vi "fn Browse Server.vi"(8 "error in (no error)":errorcluster) -> (0 "error out":errorcluster, 3 "[Items]":string[](array[string]))   [LabVIEW 2018, in "LV_OPC.lvlib"]
doc: "LVOPC_API int fnBrowseServer(char* LV_items[]);"
uses:
  LV_OPC.lvlib
  LVOPC64.dll
panel:
  out "LV_items out":string
  out "function return":i32
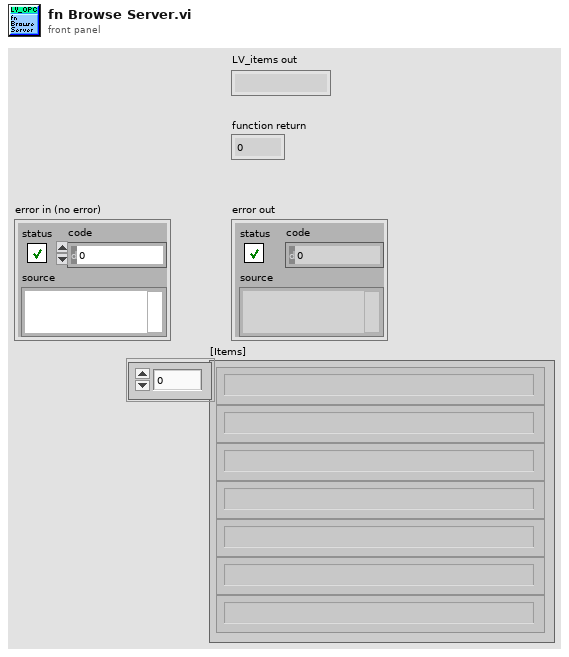
[diagram p1: front panel]
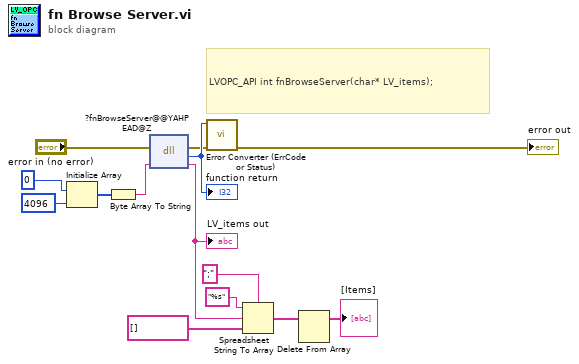
[diagram p0: block diagram]
diagram:
  # "LVOPC_API int fnBrowseServer(char* LV_items);"
  n1 = Initialize Array(u8 0 ("element"), 4096 ("dimension size")) -> (w8:u8[])
  n2 = Byte Array To String(unsigned byte array=w8) -> (string=w7:string)
  n3 = dll-call lib="C:/Users/Andrey/Desktop/LV_OPC-Client-x64/LV_OPC_Test/OPC.DLL/LVOPC64.*" fn="?fnBrowseServer@@YAHPEAD@Z"(error in="error in (no error)", "LV_items"=w7) -> (error out=w12:errorcluster, "return type"=w14:i32, "LV_items"=w1:string)  [unwired: 2 in, 1 out]
  "function return" <- w14
  "LV_items out" <- w1
  n4 = call "Error Converter (ErrCode or Status).vi"("error in (no error)"=w12, "error code"=w14) -> ("error out"=→"error out":errorcluster)  [unwired: 9 in]
  n5 = Spreadsheet String To Array(delimiter (Tab)=";", format string="%s", spreadsheet string=w1, array type (2D Dbl)=string[] []) -> (array=w3:string[])
  n6 = Delete From Array(array=w3) -> (array with subset deleted=→"[Items]":string[])  [unwired: 2 in, 1 out]
